vi "DraggingDresser.vi"() -> ()   [LabVIEW 2015]
panel:
  out "Force":dbl[](array[numeric])
  out "Angle for Minimum Force":i32 format="%.1f"
  in  "Coefficient of Kinetic Friction":dbl format="%.1f"
  out "Waveform Graph":dbl[](graph)
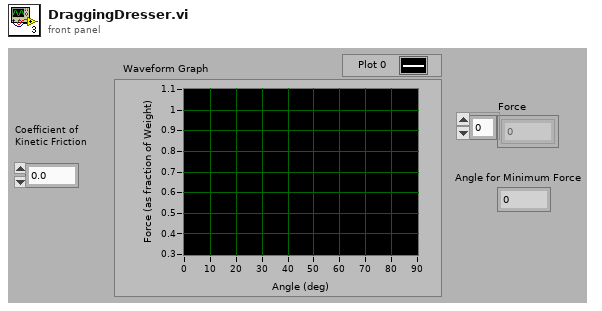
[diagram p1: front panel]
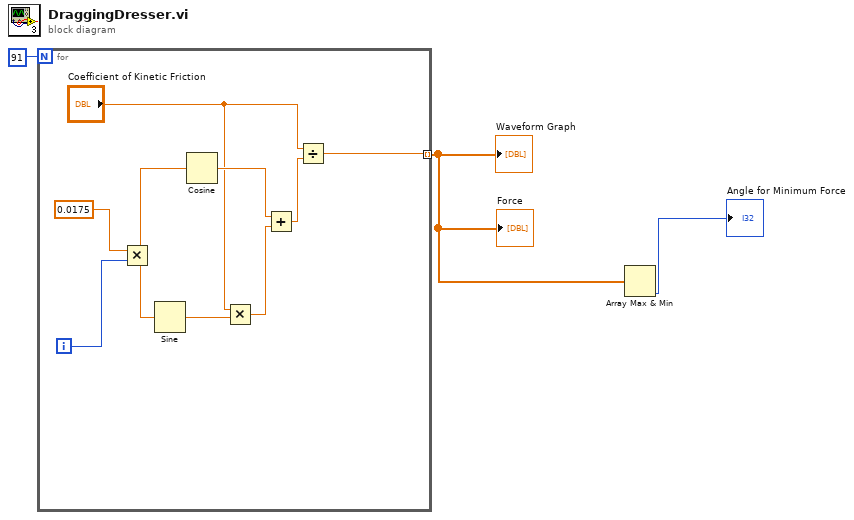
[diagram p0: block diagram]
diagram:
  n1 = for {
    N: 91 -> [_]
    tunnel: [w7] -> w1 mode=indexing
    i -> [w12]
    n2 = Multiply(x=0.0175, y=w12) -> (x*y=w10:dbl)
    n3 = Sine(x=w10) -> (sin(x)=w5:dbl)
    n4 = Cosine(x=w10) -> (cos(x)=w9:dbl)
    n5 = Multiply(x="Coefficient of Kinetic Friction", y=w5) -> (x*y=w4:dbl)
    n6 = Add(x=w9, y=w4) -> (x+y=w8:dbl)
    n7 = Divide(x="Coefficient of Kinetic Friction", y=w8) -> (x/y=w7:dbl)
  }
  "Force" <- w1
  "Waveform Graph" <- w1
  n8 = Array Max & Min(array=w1) -> (min index (indices)=→"Angle for Minimum Force":i32)  [unwired: 3 out]
